vi "VFH-convert_Excel.vi"() -> ()   [LabVIEW 2020, in "VFH-VNA_File_Handler.lvlib"]
uses:
  VFH-VNA_File_Handler.lvlib
  <userlib>/_OpenG.lib/file/file.llb/openg_file.lvlib
panel:
  out "error out":errorcluster
  out "All Files in Dir":path[](array[path])
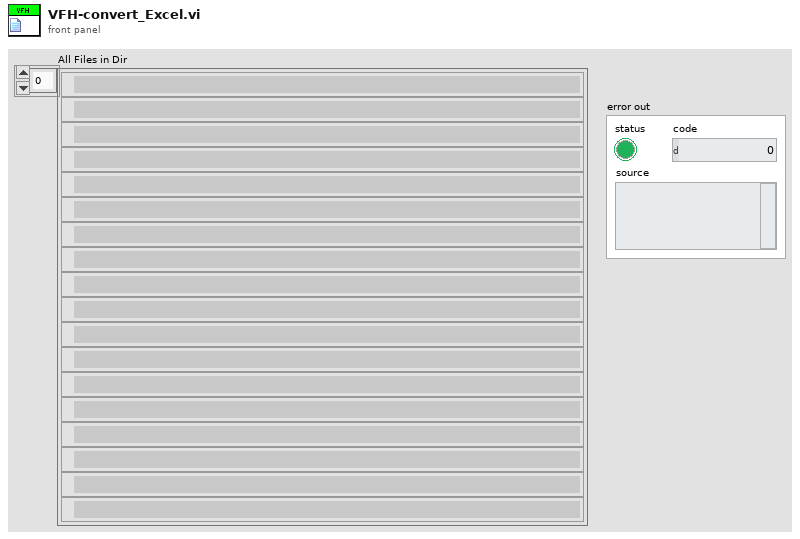
[diagram p1: front panel]
types:
  T1 = typedef "VFH-VNA_File_Handler.lvlib/VFH-file_cluster-NanoVNA.ctl" = cluster{"Frequency":dbl[], "S11_Real":dbl[], "S11_Imag":dbl[], "S21_Real":dbl[], "S21_Imag":dbl[], "S12_Real":dbl[], "S12_Imag":dbl[], "S22_Real":dbl[], "S22_Imag":dbl[]}
  T2 = typedef "VFH-VNA_File_Handler.lvlib/VFH-file_cluster-r140.ctl" = cluster{"Frequency":dbl[], "Permativity'":dbl[], "Permativity''":dbl[], "Q [S/m]":dbl[], "Tan":dbl[], "Reflection R":dbl[], "Reflection I":dbl[]}
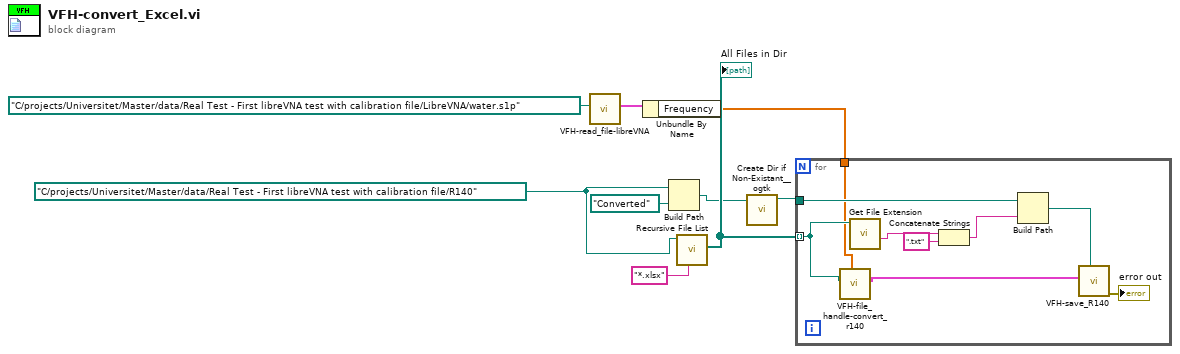
[diagram p0: block diagram]
diagram:
  w7 = path "C:/projects/Universitet/Master/data/Real Test - First libreVNA test with calibration file/R140" ("Folder Path")
  n1 = call "VFH-read_file-libreVNA.vi"("file path (dialog if empty)"=path "C:/projects/Universitet/Master/data/Real Test - First libreVNA test with calibration file/LibreVNA/water.s1p") -> ("output cluster"=w2:T1)  [unwired: 9 in, 1 out]
  n2 = Unbundle By Name(w2) -> ("Frequency"=w1:dbl[])
  n3 = Build Path(base path=w7, name or relative path=path "Converted") -> (appended path=w5:path)
  n4 = call <vilib>:"Recursive File List.vi"("pattern"="*.xlsx", "Folder Path"=w7) -> ("All Files in Dir"=w8:path[])  [unwired: 5 in, 4 out]
  "All Files in Dir" <- w8
  n5 = call <userlib>:"Create Dir if Non-Existant__ogtk.vi"("Directory Path"=w5) -> ("dup Directory Path"=w4:path)  [unwired: 8 in, 2 out]
  n6 = for {
    tunnel: w8 -> [w12] mode=indexing
    tunnel: w4 -> [w15]
    tunnel: w1 -> [w10]
    n7 = call "VFH-file_handle-convert_r140.vi"("Xi"=w10, "file path (dialog if empty)"=w12) -> ("Handled data"=w11:T2)  [unwired: 9 in]
    n8 = call <vilib>:"Get File Extension.vi"("file"=w12) -> ("filename without extension"=w18:string)  [unwired: 6 in, 4 out]
    n9 = Concatenate Strings(w18, ".txt" ("string")) -> (w16:string)
    n10 = Build Path(base path=w15, name or relative path=w16) -> (appended path=w14:path)
    n11 = call "VFH-save_R140.vi"("file path (use dialog)"=w14, "input"=w11) -> ("error out"=→"error out":errorcluster)  [unwired: 9 in]
  }
